vi "Get Value (String).vi"(8 "error in (no error)":errorcluster, 10 "key":string, 11 "JSON Object in":refnum<class "JSON Object.lvclass">) -> (0 "error out":errorcluster, 1 "found":bool, 2 "value":refnum<class "JSON String.lvclass">)   [LabVIEW 2015, in "LVJSON.lvlib" / "JSON Object.lvclass"]
uses:
  JSON Object.lvclass
  JSON String/JSON String.lvclass
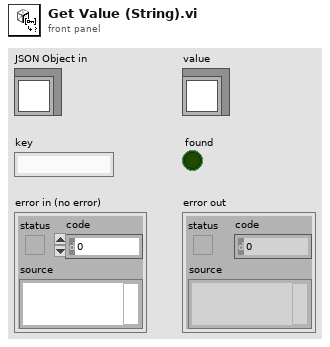
[diagram p1: front panel]
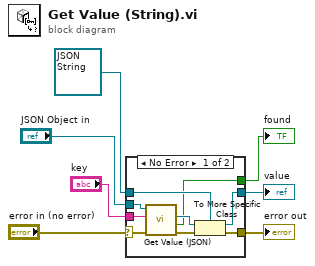
[diagram p0: block diagram]
diagram:
  n1 = case shown="No Error" "error in (no error)" {
    selector: "error in (no error)" -> [w14 w18]
    tunnel: [w10 w18] -> w6
    tunnel: "JSON Object in" -> [w16 _]
    tunnel: "key" -> [w15 _]
    tunnel: [w12 w17] -> w2
    tunnel: refnum<class "JSON String.lvclass"> refnum ("JSON String.lvclass") -> [w9 w17]
    tunnel: [w8 _] -> w1
    frame No Error {
      n2 = call "Get Value (JSON).vi"("error in (no error)"=w14, "key"=w15, "JSON Object in"=w16) -> ("error out"=w11:errorcluster, "found"=w8:bool, "value"=w13:refnum<class "JSON Datatype.lvclass">)  [unwired: 6 in]
      n3 = To More Specific Class(target class=w9, reference=w13, error in=w11) -> (specific class reference=w12:refnum<class "JSON String.lvclass">, error out=w10:errorcluster)
    }
    frame Error {
    }
  }
  "error out" <- w6
  "value" <- w2
  "found" <- w1
